vi "Update Setting.vi"(6 "Update Setting:":T1, 8 "error in":errorcluster, 11 "DMK33UP2000 in":refnum<class "DMK33UP2000.lvclass">) -> (0 "error out":errorcluster, 2 "Supported?":bool, 3 "DMK33UP2000 out":refnum<class "DMK33UP2000.lvclass">)   [LabVIEW 2018, in "DMK33UP2000.lvlib" / "DMK33UP2000.lvclass"]
uses:
  DMK33UP2000.lvclass
  builds/Camera.lvlibp/Custom Controls/Camera Setting.ctl
  builds/Camera.lvlibp/Camera.lvclass
  <vilib>/vision/driver/NI_Vision_Acquisition_Software.lvlib
  C:/Users/Ron.Dexter.LUMINARTECH/Desktop/builds/Camera.lvlibp/Camera.lvclass
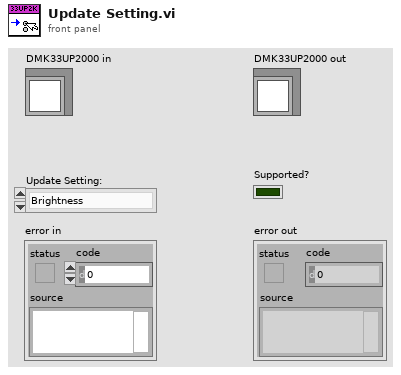
[diagram p1: front panel]
types:
  T1 = typedef "Camera.lvlibp/Camera.lvclass/Camera Setting.ctl" = enum16{"Brightness", "Rotation", "Contrast", "Exposure", "Frame Rate", "Gain", "Gamma", "Image Resolution", "Sharpness"}
  T2 = typedef "Camera.lvlibp/IMAQdx.ctl" = refnum<k21>
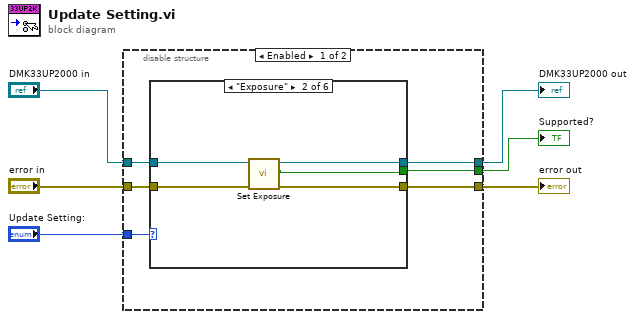
[diagram p0: block diagram]
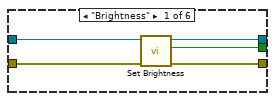
[diagram p2: hidden frame]
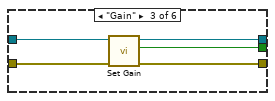
[diagram p3: hidden frame]
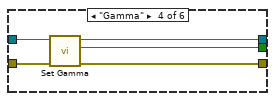
[diagram p4: hidden frame]
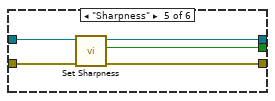
[diagram p5: hidden frame]
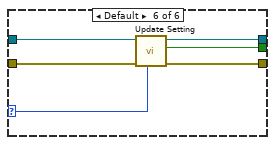
[diagram p6: hidden frame]
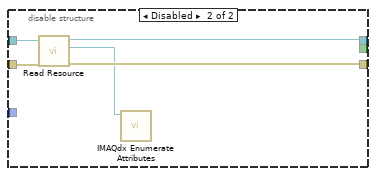
[diagram p7: hidden frame]
diagram:
  n1 = disable-structure shown="Enabled" {
    disable-tunnel: [w12 w45] -> w6
    disable-tunnel: [w11 _] -> w5
    disable-tunnel: [w10 w46] -> w4
    disable-tunnel: "error in" -> [w9 w47]
    disable-tunnel: "DMK33UP2000 in" -> [w8 w48]
    disable-tunnel: "Update Setting:" -> [w7 _]
    frame Enabled {
      n2 = case shown="\"Exposure\"" w7 {
        selector: w7 -> [_ _ _ _ _ w38]
        tunnel: [w14 w19 w24 w28 w35 w43] -> w12
        tunnel: [w13 w18 w23 w29 w33 w42] -> w11
        tunnel: [w15 w21 w25 w30 w34 w41] -> w10
        tunnel: w9 -> [w16 w20 w26 w31 w36 w40]
        tunnel: w8 -> [w17 w22 w27 w32 w37 w39]
        frame "Brightness" {
          n3 = call "Set Brightness.vi"("error in"=w16, "DMK33UP2000 in"=w17) -> ("error out"=w14:errorcluster, "Supported?"=w13:bool, "DMK33UP2000 out"=w15:refnum<class "DMK33UP2000.lvclass">)  [unwired: 7 in]
        }
        frame "Exposure" {
          n4 = call "Set Exposure.vi"("error in"=w20, "DMK33UP2000 in"=w22) -> ("error out"=w19:errorcluster, "Supported?"=w18:bool, "DMK33UP2000 out"=w21:refnum<class "DMK33UP2000.lvclass">)  [unwired: 7 in]
        }
        frame "Gain" {
          n5 = call "Set Gain.vi"("error in"=w26, "DMK33UP2000 in"=w27) -> ("error out"=w24:errorcluster, "Supported?"=w23:bool, "DMK33UP2000 out"=w25:refnum<class "DMK33UP2000.lvclass">)  [unwired: 7 in]
        }
        frame "Gamma" {
          n6 = call "Set Gamma.vi"("error in"=w31, "DMK33UP2000 in"=w32) -> ("error out"=w28:errorcluster, "Supported?"=w29:bool, "DMK33UP2000 out"=w30:refnum<class "DMK33UP2000.lvclass">)  [unwired: 7 in]
        }
        frame "Sharpness" {
          n7 = call "Set Sharpness.vi"("error in"=w36, "DMK33UP2000 in"=w37) -> ("error out"=w35:errorcluster, "Supported?"=w33:bool, "DMK33UP2000 out"=w34:refnum<class "DMK33UP2000.lvclass">)  [unwired: 7 in]
        }
        frame Default {
          n8 = call-parent "Update Setting.vi"("Update Setting:"=w38, "error in"=w40, "Camera in"=w39) -> ("error out"=w43:errorcluster, "Supported?"=w42:bool, "Camera out"=w41:refnum<class "DMK33UP2000.lvclass">)  [unwired: 6 in]
        }
      }
    }
    frame Disabled {
      n9 = call "Read Resource.vi"("error in (no error)"=w47, "Camera in"=w48) -> ("error out"=w45:errorcluster, "IMAQdx Session"=w44:T2, "Camera out"=w46:refnum<class "DMK33UP2000.lvclass">)  [unwired: 7 in]
      n10 = call <vilib>:"IMAQdx Enumerate Attributes.vi"("Session In"=w44) -> ()  [unwired: 8 in, 3 out]
    }
  }
  "error out" <- w6
  "DMK33UP2000 out" <- w4
  "Supported?" <- w5
